vi "Read Controller Enqueuer.vi"(11 "冷却器":refnum<class "Cooler.lvclass">) -> (2 "控制器待入队列":refnum<class "Message Enqueuer.lvclass">)   [LabVIEW 2015, in "Cooler.lvlib" / "Cooler.lvclass"]
doc: "读取向控制器操作者发送消息的待入队列。由于冷却器当前可能不受任何控制器的控制，该VI可能返回“非法引用句柄”待入队列。"
uses:
  Cooler.lvclass
  <vilib>/ActorFramework/Message Enqueuer/Message Enqueuer.lvclass
  Cooler.lvclass/Cooler.ctl
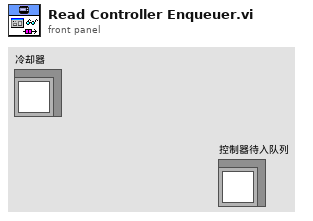
[diagram p1: front panel]
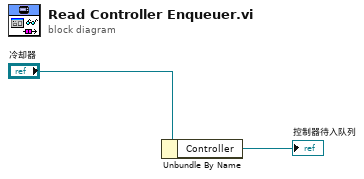
[diagram p0: block diagram]
diagram:
  n1 = Unbundle By Name("冷却器") -> ("Controller"=→"控制器待入队列":refnum<class "Message Enqueuer.lvclass">)
